vi "Test_DSP1500-30WE_visa-raw.vi"() -> ()   [LabVIEW 2019]
uses:
  <vilib>/Instr/_visa.llb/VISA Open Access Mode.ctl
panel:
  out "길이":i32=33
  out "read buffer":string="iDRC,DSP1500-30WE,702648,1.03.42\n"
  out "error out":errorcluster
  in  "VISA":refnum<visa-resource-name>="TCPIP0::192.168.0.14::HISLIP0::INSTR"
  in  "Byte count":u32=33
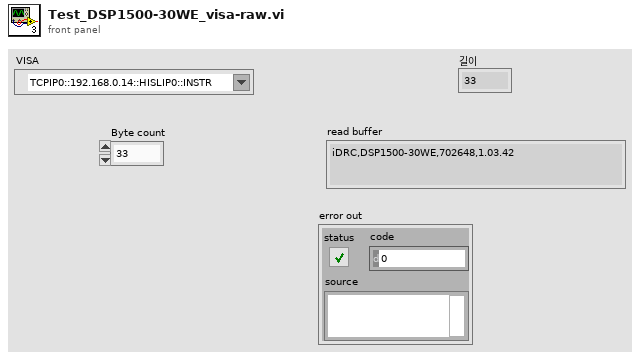
[diagram p1: front panel]
types:
  T1 = typedef "VISA Open Access Mode.ctl" = u32
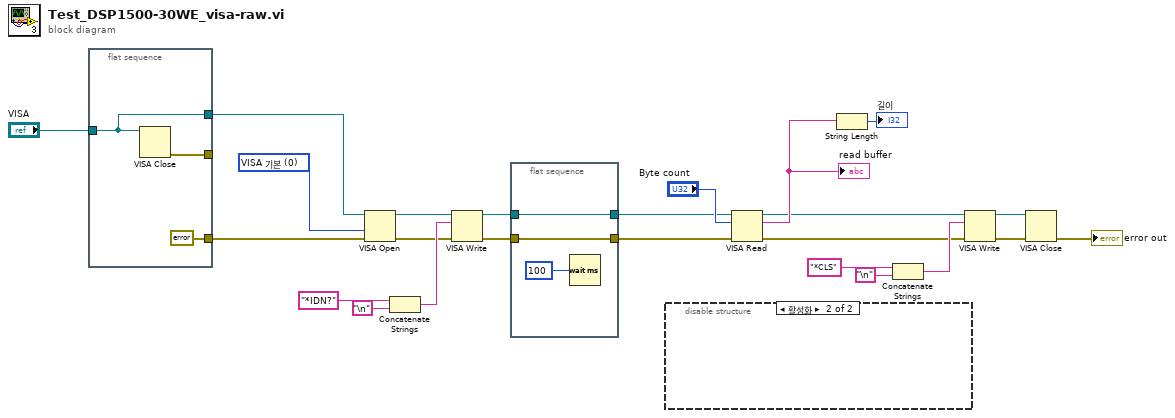
[diagram p0: block diagram]
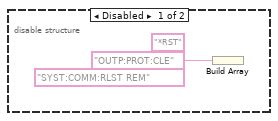
[diagram p2: hidden frame]
diagram:
  w17 = T1 0 items=["VISA 기본"=0, "배타적인 잠금"=1, "설정된 셋팅 로드"=4] ("Access Mode")
  n1 = flat-sequence {
    tunnel: "VISA" -> [w25]
    tunnel: [w27] -> _
    tunnel: [errorcluster {"status"=FALSE, "code"=0, "source"=""} ("에러 입력(에러 없음)")] -> w10
    tunnel: [w25] -> w9
    frame #0 {
      n2 = VISA Close(VISA resource name=w25) -> (error out=w27:errorcluster)  [unwired: 1 in]
    }
  }
  n3 = VISA Open(access mode=w17, error in (no error)=w10, VISA resource name=w9) -> (VISA resource name=w16:refnum<visa-resource-name>, error out=w14:errorcluster)  [unwired: 2 in]
  n4 = Concatenate Strings("*IDN?" ("Command"), "\n") -> (w19:string)
  n5 = VISA Write(VISA resource name=w16, write buffer=w19, error in (no error)=w14) -> (VISA resource name out=w23:refnum<visa-resource-name>, error out=w22:errorcluster)  [unwired: 1 out]
  n6 = flat-sequence {
    tunnel: w23 -> [w30]
    tunnel: w22 -> [w29]
    tunnel: [w30] -> w21
    tunnel: [w29] -> w20
    frame #0 {
      n7 = Wait (ms)(milliseconds to wait=u32 100 ("대기 시간 (ms)")) -> ()  [unwired: 1 out]
    }
  }
  n8 = disable-structure shown="활성화" {
    frame Disabled {
      (unwired) "*RST" ("Command")
      (unwired) "SYST:COMM:RLST REM"
      n9 = Build Array("OUTP:PROT:CLE" ("Command")) -> ()  [unwired: 1 out]
    }
    frame Enabled {
    }
  }
  n10 = VISA Read(VISA resource name=w21, byte count="Byte count", error in (no error)=w20) -> (VISA resource name out=w5:refnum<visa-resource-name>, read buffer=w13:string, error out=w4:errorcluster)  [unwired: 1 out]
  "read buffer" <- w13
  n11 = String Length(string=w13) -> (length=→"길이":i32)
  n12 = Concatenate Strings("*CLS" ("Command"), "\n") -> (w6:string)
  n13 = VISA Write(VISA resource name=w5, write buffer=w6, error in (no error)=w4) -> (VISA resource name out=w3:refnum<visa-resource-name>, error out=w2:errorcluster)  [unwired: 1 out]
  n14 = VISA Close(VISA resource name=w3, error in (no error)=w2) -> (error out=→"error out":errorcluster)
